vi "KeyDownLightKeyUpOff.vi"() -> ()   [LabVIEW 2015]
uses:
  <vilib>/Utility/inputDevices.llb/keyboardAcquire.vi
panel:
  out "error out":errorcluster
  in  "task/channels in":refnum<k21>
  in  "Stop Button":bool
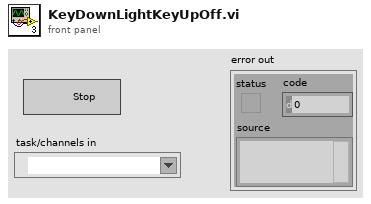
[diagram p1: front panel]
types:
  T1 = enum16{"0", "1", "2", "3", "4", "5", "6", "7", "8", "9", "A", "B", "C", "D", "E", "F", "G", "H", "I", "J", "K", "L", "M", "N", "O", "P", "Q", "R", "S", "T", "U", "V", "W", "X", "Y", "Z", "F1", "F2", "F3", "F4", "F5", "F6", "F7", "F8", "F9", "F10", "F11", "F12", "F13", "F14", "F15", "ADD", "BACK", "BACKSLASH", "CAPITAL", "COMMA", "DECIMAL", "DELETE", "DIVIDE", "DOWN", "END", "EQUALS", "ESCAPE", "GRAVE (`)", "HOME", "INSERT", "LBRACKET", "LCONTROL", "LEFT", "L ALT", "LSHIFT", "LWIN", "MINUS", "MULTIPLY", "NEXT", "NUMLOCK", "NUMPAD_0", "NUMPAD_1", "NUMPAD_2", "NUMPAD_3", "NUMPAD_4", "NUMPAD_5", "NUMPAD_6", "NUMPAD_7", "NUMPAD_8", "NUMPAD_9", "PAUSE", "PERIOD", "PRIOR (PG UP)", "RBRACKET", "RCONTROL", "RETURN", "RIGHT", "R ALT", "RSHIFT", "RWIN", "SCROLL", "SEMICOLON", "SLASH", "SPACE", "SUBTRACT", "TAB", "UP", "ENTER (num pad)", "' (quote)"}[]
  T2 = enum16{"0", "1", "2", "3", "4", "5", "6", "7", "8", "9", "A", "B", "C", "D", "E", "F", "G", "H", "I", "J", "K", "L", "M", "N", "O", "P", "Q", "R", "S", "T", "U", "V", "W", "X", "Y", "Z", "F1", "F2", "F3", "F4", "F5", "F6", "F7", "F8", "F9", "F10", "F11", "F12", "F13", "F14", "F15", "ADD", "BACK", "BACKSLASH", "CAPITAL", "COMMA", "DECIMAL", "DELETE", "DIVIDE", "DOWN", "END", "EQUALS", "ESCAPE", "GRAVE (`)", "HOME", "INSERT", "LBRACKET", "LCONTROL", "LEFT", "L ALT", "LSHIFT", "LWIN", "MINUS", "MULTIPLY", "NEXT", "NUMLOCK", "NUMPAD_0", "NUMPAD_1", "NUMPAD_2", "NUMPAD_3", "NUMPAD_4", "NUMPAD_5", "NUMPAD_6", "NUMPAD_7", "NUMPAD_8", "NUMPAD_9", "PAUSE", "PERIOD", "PRIOR (PG UP)", "RBRACKET", "RCONTROL", "RETURN", "RIGHT", "R ALT", "RSHIFT", "RWIN", "SCROLL", "SEMICOLON", "SLASH", "SPACE", "SUBTRACT", "TAB", "UP", "ENTER (num pad)", "' (quote)"}
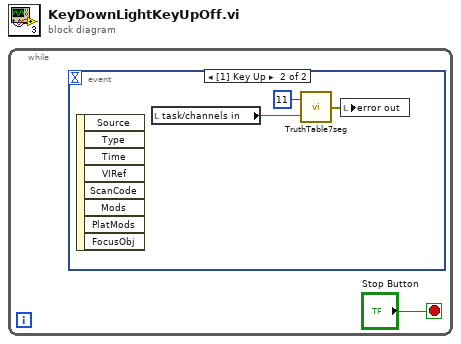
[diagram p0: block diagram]
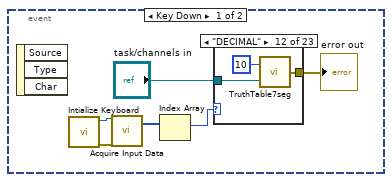
[diagram p2: hidden frame]
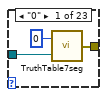
[diagram p3: hidden frame]
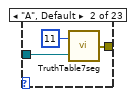
[diagram p4: hidden frame]
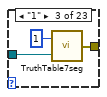
[diagram p5: hidden frame]
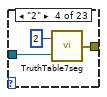
[diagram p6: hidden frame]
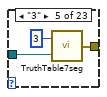
[diagram p7: hidden frame]
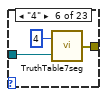
[diagram p8: hidden frame]
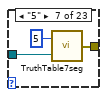
[diagram p9: hidden frame]
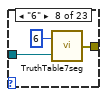
[diagram p10: hidden frame]
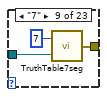
[diagram p11: hidden frame]
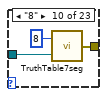
[diagram p12: hidden frame]
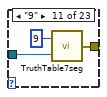
[diagram p13: hidden frame]
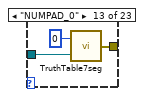
[diagram p14: hidden frame]
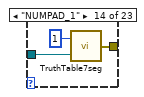
[diagram p15: hidden frame]
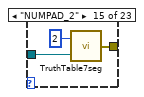
[diagram p16: hidden frame]
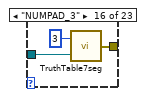
[diagram p17: hidden frame]
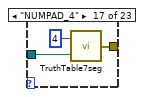
[diagram p18: hidden frame]
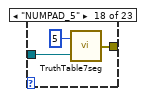
[diagram p19: hidden frame]
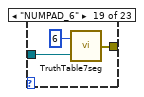
[diagram p20: hidden frame]
diagram:
  n1 = while {
    stop <- "Stop Button" stop-if-true
    n2 = event shown="[1] Key Up" {
      selector: _ -> [_ _]
      dyn-events: _ -> [_ _]
      timeout: _ -> [_ _]
      event Key Down {
        n3 = event-data() -> ()  [unwired: 1 in, 3 out]
        n4 = call <vilib>:"Intialize Keyboard.vi"() -> ("error out"=w5:errorcluster, "device ID"=w4:refnum<k1>)  [unwired: 10 in]
        n5 = call-poly <vilib>:"Acquire Input Data.vi"("device ID"=w4, "error in (no error)"=w5) -> ("keys pressed"=w6:T1)  [unwired: 15 in, 2 out]
        n6 = Index Array(array=w6) -> (element=w2:T2)  [unwired: 1 in]
        n7 = case shown="\"DECIMAL\"" w2 {
          tunnel: [w9 w11 w15 w18 w20 w23 w26 w29 w32 w35 w38 w42 w44 w47 w50 w53 w56 w59 w62 w65 w68 w71 w74] -> w7
          tunnel: "task/channels in" -> [w8 w12 w14 w17 w21 w24 w27 w30 w33 w36 w39 w41 w45 w48 w51 w54 w57 w60 w63 w66 w69 w72 w75]
          frame "0" {
            n8 = call "TruthTable7seg.vi"("task/channels in"=w8, "Numeric Control"=0) -> ("error out 2"=w9:errorcluster)
          }
          frame "A", Default {
            n9 = call "TruthTable7seg.vi"("task/channels in"=w12, "Numeric Control"=11) -> ("error out 2"=w11:errorcluster)
          }
          frame "1" {
            n10 = call "TruthTable7seg.vi"("task/channels in"=w14, "Numeric Control"=1) -> ("error out 2"=w15:errorcluster)
          }
          frame "2" {
            n11 = call "TruthTable7seg.vi"("task/channels in"=w17, "Numeric Control"=2) -> ("error out 2"=w18:errorcluster)
          }
          frame "3" {
            n12 = call "TruthTable7seg.vi"("task/channels in"=w21, "Numeric Control"=3) -> ("error out 2"=w20:errorcluster)
          }
          frame "4" {
            n13 = call "TruthTable7seg.vi"("task/channels in"=w24, "Numeric Control"=4) -> ("error out 2"=w23:errorcluster)
          }
          frame "5" {
            n14 = call "TruthTable7seg.vi"("task/channels in"=w27, "Numeric Control"=5) -> ("error out 2"=w26:errorcluster)
          }
          frame "6" {
            n15 = call "TruthTable7seg.vi"("task/channels in"=w30, "Numeric Control"=6) -> ("error out 2"=w29:errorcluster)
          }
          frame "7" {
            n16 = call "TruthTable7seg.vi"("task/channels in"=w33, "Numeric Control"=7) -> ("error out 2"=w32:errorcluster)
          }
          frame "8" {
            n17 = call "TruthTable7seg.vi"("task/channels in"=w36, "Numeric Control"=8) -> ("error out 2"=w35:errorcluster)
          }
          frame "9" {
            n18 = call "TruthTable7seg.vi"("task/channels in"=w39, "Numeric Control"=9) -> ("error out 2"=w38:errorcluster)
          }
          frame "DECIMAL" {
            n19 = call "TruthTable7seg.vi"("task/channels in"=w41, "Numeric Control"=10) -> ("error out 2"=w42:errorcluster)
          }
          frame "NUMPAD_0" {
            n20 = call "TruthTable7seg.vi"("task/channels in"=w45, "Numeric Control"=0) -> ("error out 2"=w44:errorcluster)
          }
          frame "NUMPAD_1" {
            n21 = call "TruthTable7seg.vi"("task/channels in"=w48, "Numeric Control"=1) -> ("error out 2"=w47:errorcluster)
          }
          frame "NUMPAD_2" {
            n22 = call "TruthTable7seg.vi"("task/channels in"=w51, "Numeric Control"=2) -> ("error out 2"=w50:errorcluster)
          }
          frame "NUMPAD_3" {
            n23 = call "TruthTable7seg.vi"("task/channels in"=w54, "Numeric Control"=3) -> ("error out 2"=w53:errorcluster)
          }
          frame "NUMPAD_4" {
            n24 = call "TruthTable7seg.vi"("task/channels in"=w57, "Numeric Control"=4) -> ("error out 2"=w56:errorcluster)
          }
          frame "NUMPAD_5" {
            n25 = call "TruthTable7seg.vi"("task/channels in"=w60, "Numeric Control"=5) -> ("error out 2"=w59:errorcluster)
          }
          frame "NUMPAD_6" {
            n26 = call "TruthTable7seg.vi"("task/channels in"=w63, "Numeric Control"=6) -> ("error out 2"=w62:errorcluster)
          }
          frame "NUMPAD_7" {
            n27 = call "TruthTable7seg.vi"("task/channels in"=w66, "Numeric Control"=7) -> ("error out 2"=w65:errorcluster)
          }
          frame "NUMPAD_8" {
            n28 = call "TruthTable7seg.vi"("task/channels in"=w69, "Numeric Control"=8) -> ("error out 2"=w68:errorcluster)
          }
          frame "NUMPAD_9" {
            n29 = call "TruthTable7seg.vi"("task/channels in"=w72, "Numeric Control"=9) -> ("error out 2"=w71:errorcluster)
          }
          frame "PERIOD" {
            n30 = call "TruthTable7seg.vi"("task/channels in"=w75, "Numeric Control"=10) -> ("error out 2"=w74:errorcluster)
          }
        }
        "error out" <- w7
      }
      event Key Up {
        n31 = event-data() -> ()  [unwired: 1 in, 8 out]
        n32 = local read "task/channels in"() -> (w79:refnum<k21>)
        n33 = call "TruthTable7seg.vi"("task/channels in"=w79, "Numeric Control"=11) -> ("error out 2"=w77:errorcluster)
        n34 = local write "error out"(w77) -> ()
      }
    }
  }
